vi "LWXPS_ControllerMotionKernelPeriodMinMaxGet.vi"(1 "XPS Reference IN":refnum<k24>, 4 "LabVIEW error IN":errorcluster) -> (10 "XPS Reference OUT":refnum<k24>, 11 "LabVIEW error OUT":errorcluster, 12 "Returned error code":i32, 13 "XPS Error String":string, 14 "Minimum Corrector Period":dbl, 15 "Maximum Corrector Period":dbl, 16 "Minimum Profiler Period":dbl, 17 "Maximum Profiler Period":dbl, 18 "Minimum Servitudes Period":dbl, 19 "Maximum Servitudes Period":dbl)   [LabVIEW 2014]
uses:
  D:/XPSQ8_LabView_Library/Development/Source/Dll/Newport.XPS.CommandInterface.dll
  Dll/Newport.XPS.CommandInterface.dll
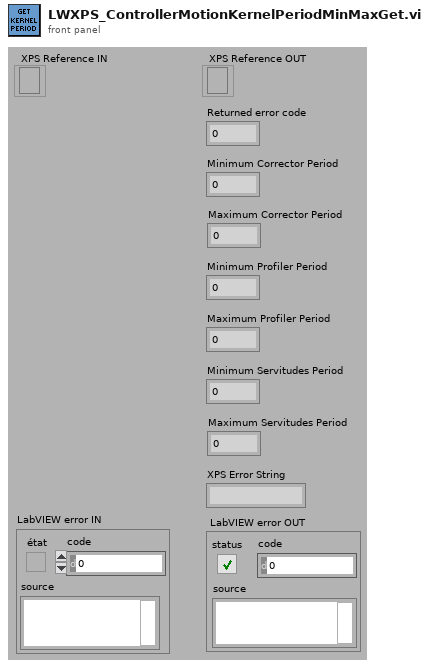
[diagram p1: front panel]
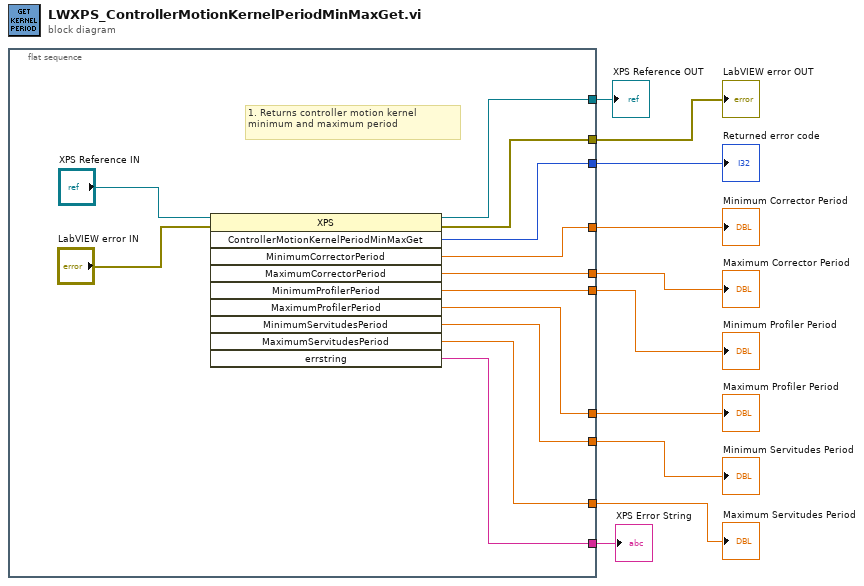
[diagram p0: block diagram]
diagram:
  n1 = flat-sequence {
    tunnel: [w19] -> w9
    tunnel: [w20] -> w10
    tunnel: [w18] -> w8
    tunnel: [w13] -> w7
    tunnel: [w17] -> w6
    tunnel: [w15] -> w4
    tunnel: [w11] -> w2
    tunnel: [w14] -> w3
    tunnel: [w12] -> w1
    tunnel: [w16] -> w5
    frame #0 {
      # "1. Returns controller motion kernel minimum and maximum period"
      n2 = invoke class="XPS" method="ControllerMotionKernelPeriodMinMaxGet"(reference="XPS Reference IN", error in="LabVIEW error IN") -> (reference out=w19:refnum<k24>, error out=w20:errorcluster, "ControllerMotionKernelPeriodMinMaxGet"=w18:i32, "MinimumCorrectorPeriod"=w13:dbl, "MaximumCorrectorPeriod"=w17:dbl, "MinimumProfilerPeriod"=w16:dbl, "MaximumProfilerPeriod"=w15:dbl, "MinimumServitudesPeriod"=w14:dbl, "MaximumServitudesPeriod"=w12:dbl, "errstring"=w11:string)  [unwired: 8 in]
    }
  }
  "XPS Reference OUT" <- w9
  "LabVIEW error OUT" <- w10
  "Returned error code" <- w8
  "Minimum Corrector Period" <- w7
  "Maximum Corrector Period" <- w6
  "Minimum Profiler Period" <- w5
  "Maximum Profiler Period" <- w4
  "Minimum Servitudes Period" <- w3
  "Maximum Servitudes Period" <- w1
  "XPS Error String" <- w2
